vi "Run Target VI.vi"(6 "clone#":i32, 8 "doneRef":refnum<vi>, 11 "targetVIref":T1) -> ()   [LabVIEW 2020, in "NI_TargetHelper.lvlib"]
uses:
  <vilib>/TargetSupport/NI_TargetHelper/NI_TargetHelper.lvlib
  <vilib>/TargetSupport/NI_TargetHelper/Instance VIref.ctl
  761217ef-e074-c54f-a090-1f88087bb986.vi
panel:
  out "error out":errorcluster
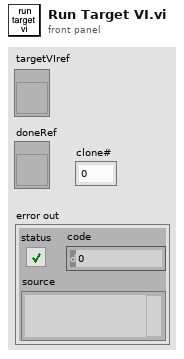
[diagram p1: front panel]
types:
  T1 = typedef "NI_TargetHelper.lvlib/Instance VIref.ctl" = refnum<vi>
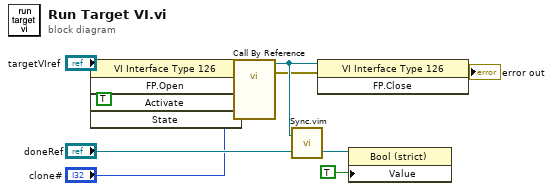
[diagram p0: block diagram]
diagram:
  n1 = invoke class="VI Interface Type 126" method="FP.Open"(reference="targetVIref", "Activate"=TRUE ("Activate?")) -> (reference out=w9:T1, error out=w3:errorcluster)  [unwired: 3 in, 3 out]
  n2 = call-by-ref "?"(reference=w9, error in=w3, "clone#"="clone#") -> (reference out=w4:T1, error out=w2:errorcluster)  [unwired: 3 in]
  n3 = call "Sync.vim"("a"=w4, "b"="doneRef") -> ("b'"=w6:refnum<vi>)  [unwired: 24 in, 1 out]
  n4 = invoke class="VI Interface Type 126" method="FP.Close"(reference=w4, error in=w2) -> (error out=→"error out":errorcluster)  [unwired: 1 in, 2 out]
  n5 = property class="Bool (strict)"(reference=w6, "Value"=TRUE) -> ()  [unwired: 1 in, 2 out]
